vi "Refresh Pixel clock.vi"(8 "Pixel clock_pulse width(tick)":i32, 9 "Pixel pulse_initial delay":i32, 10 "Pixel clock_pulse width":i32, 11 "Refresh input":bool) -> (3 "Refresh output":bool)   [LabVIEW 2015]
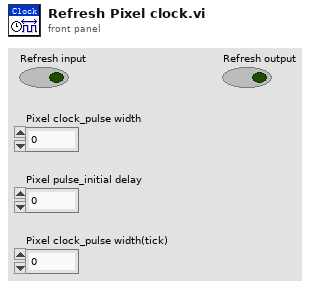
[diagram p1: front panel]
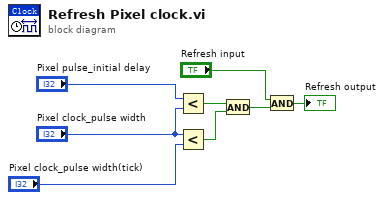
[diagram p0: block diagram]
diagram:
  n1 = Less?(x="Pixel pulse_initial delay", y="Pixel clock_pulse width") -> (x < y?=w2:bool)
  n2 = Less?(x="Pixel clock_pulse width", y="Pixel clock_pulse width(tick)") -> (x < y?=w3:bool)
  n3 = And(x=w2, y=w3) -> (x .and. y?=w5:bool)
  n4 = And(x="Refresh input", y=w5) -> (x .and. y?=→"Refresh output":bool)
